vi "ServerTake2.vi"() -> ()   [LabVIEW 2021]
uses:
  86556008-d19e-4632-a649-a7f0de4e085f.vi
  5d9f77ae-4eb7-4624-8507-499cb33e88e0.vi
  9a779ec1-8874-4ed7-8bc4-c0cd389ef899.vi
  3957625e-ef2c-40df-94d6-cc40180103aa.vi
  b28d0b89-d437-4566-8e34-c46da29a0ee1.vi
  6f342689-c146-4fba-b3a6-fb699f7c09ee.vi
  <vilib>/Utility/file.llb/Write Delimited Spreadsheet (string).vi
panel:
  in  "file path (dialog if empty)":path=path "D:/APU Stuff/Bachelor of Computer Science (Intelligent Systems) [APD2F2202CS(IS)]/Semester 1/System Programming and Computer Control [CT047-3-2-SPCC]/Assignment/SystemRedo/Zone Status Changes.csv"
  in  "stop":bool
  in  "Tamper":cluster{u32, u32}[](array[cluster])
  in  "Alarm":cluster{u32, u32}[](array[cluster])
  in  "Bypass":cluster{u32, u32}[](array[cluster])
  in  "Normal":cluster{u32, u32}[](array[cluster])
  out "Zone 6":bool
  out "Zone 5":bool
  out "Zone 4":bool
  out "Zone 3":bool
  out "Zone 2":bool
  out "Zone 1":bool
  # "Green = Normal\nRed = Alarm\nOrange = Tamper\nBlue = Bypass"
  # "Zone Status Indicators"
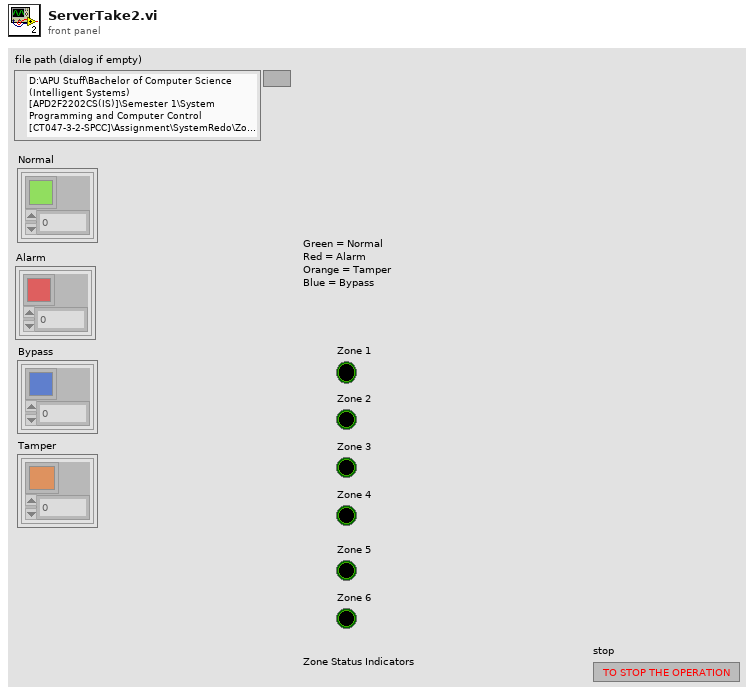
[diagram p1: front panel]
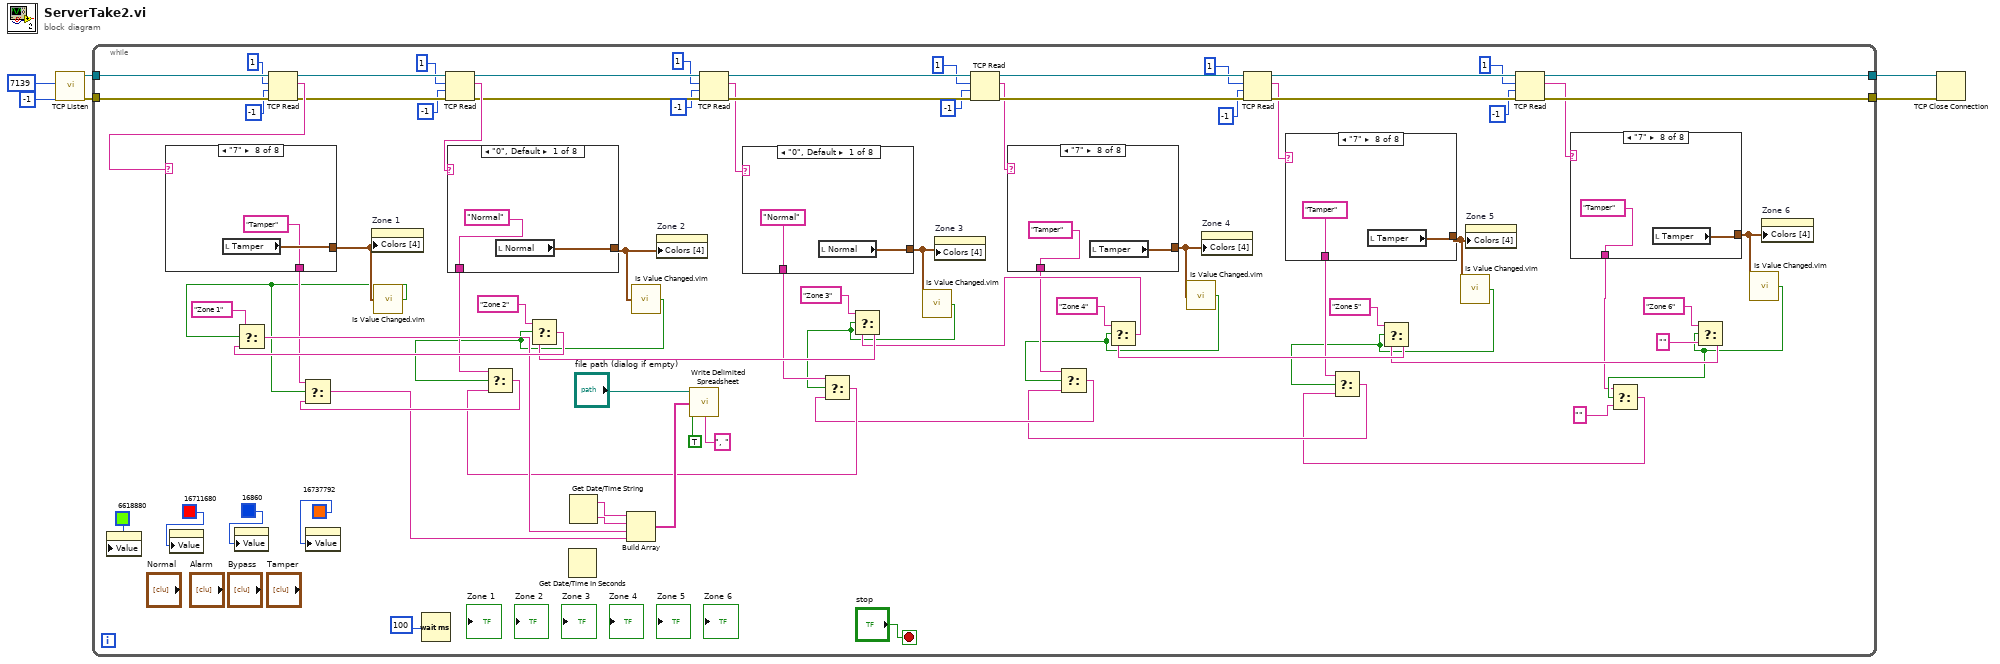
[diagram p0: block diagram]
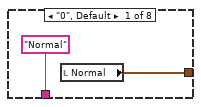
[diagram p2: hidden frame]
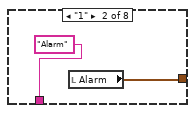
[diagram p3: hidden frame]
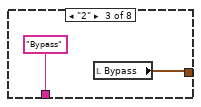
[diagram p4: hidden frame]
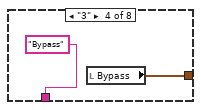
[diagram p5: hidden frame]
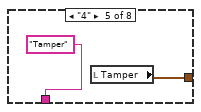
[diagram p6: hidden frame]
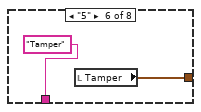
[diagram p7: hidden frame]
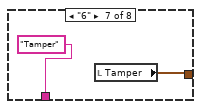
[diagram p8: hidden frame]
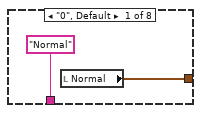
[diagram p9: hidden frame]
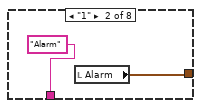
[diagram p10: hidden frame]
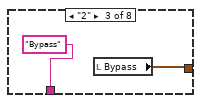
[diagram p11: hidden frame]
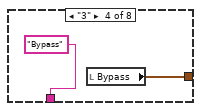
[diagram p12: hidden frame]
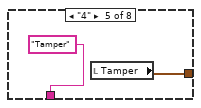
[diagram p13: hidden frame]
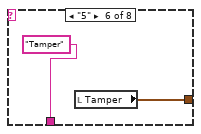
[diagram p14: hidden frame]
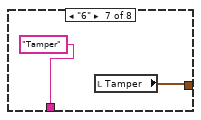
[diagram p15: hidden frame]
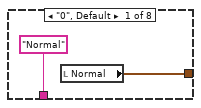
[diagram p16: hidden frame]
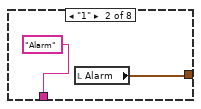
[diagram p17: hidden frame]
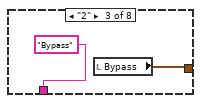
[diagram p18: hidden frame]
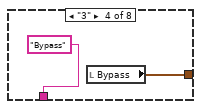
[diagram p19: hidden frame]
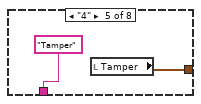
[diagram p20: hidden frame]
diagram:
  n1 = call <vilib>:"TCP Listen.vi"("timeout ms (wait forever: -1)"=-1, "port"=u16 7139) -> ("error out"=w2:errorcluster, "connection ID"=w4:refnum<k5>)  [unwired: 5 in, 3 out]
  n2 = while {
    tunnel: w4 -> [w88]
    tunnel: [w67] -> w3
    tunnel: w2 -> [w87]
    tunnel: [w63] -> w1
    stop <- "stop" stop-if-true
    n3 = property class="ColBox"("Value"=u32 6618880) -> ()  [unwired: 2 in, 2 out]
    n4 = property class="ColBox"("Value"=u32 16711680) -> ()  [unwired: 2 in, 2 out]
    n5 = property class="ColBox"("Value"=u32 16860) -> ()  [unwired: 2 in, 2 out]
    n6 = TCP Read(connection ID=w88, bytes to read=1, error in (no error)=w87, 9:-1 ("timeout ms (25000)")) -> (connection ID out=w77:refnum<k5>, data out=w84:string, error out=w76:errorcluster)  [unwired: 1 in]
    n7 = case shown="\"7\"" w84 {
      tunnel: [w170 w172 w174 w176 w178 w180 w182 w184] -> w41
      tunnel: ["Normal" "Alarm" "Bypass" "Bypass" "Tamper" "Tamper" "Tamper" "Tamper"] -> w25
      frame "0", Default {
        n8 = local read "Normal"() -> (w170:cluster{u32, u32}[])
      }
      frame "1" {
        n9 = local read "Alarm"() -> (w172:cluster{u32, u32}[])
      }
      frame "2" {
        n10 = local read "Bypass"() -> (w174:cluster{u32, u32}[])
      }
      frame "3" {
        n11 = local read "Bypass"() -> (w176:cluster{u32, u32}[])
      }
      frame "4" {
        n12 = local read "Tamper"() -> (w178:cluster{u32, u32}[])
      }
      frame "5" {
        n13 = local read "Tamper"() -> (w180:cluster{u32, u32}[])
      }
      frame "6" {
        n14 = local read "Tamper"() -> (w182:cluster{u32, u32}[])
      }
      frame "7" {
        n15 = local read "Tamper"() -> (w184:cluster{u32, u32}[])
      }
    }
    n16 = property class="ColBox"("Value"=u32 16737792) -> ()  [unwired: 2 in, 2 out]
    n17 = property on="Zone 1" class="Bool (strict)"("Colors [4]"=w41) -> ()  [unwired: 2 in, 2 out]
    n18 = call "Is Value Changed.vim"("value"=w41) -> ("changed or first call?"=w24:bool)
    n19 = Wait (ms)(milliseconds to wait=100) -> ()  [unwired: 1 out]
    n20 = TCP Read(connection ID=w77, bytes to read=1, error in (no error)=w76, 9:-1 ("timeout ms (25000)")) -> (connection ID out=w72:refnum<k5>, data out=w75:string, error out=w68:errorcluster)  [unwired: 1 in]
    n21 = case shown="\"0\", Default" w75 {
      tunnel: [w154 w156 w158 w160 w162 w164 w166 w168] -> w39
      tunnel: ["Normal" "Alarm" "Bypass" "Bypass" "Tamper" "Tamper" "Tamper" "Tamper"] -> w23
      frame "0", Default {
        n22 = local read "Normal"() -> (w154:cluster{u32, u32}[])
      }
      frame "1" {
        n23 = local read "Alarm"() -> (w156:cluster{u32, u32}[])
      }
      frame "2" {
        n24 = local read "Bypass"() -> (w158:cluster{u32, u32}[])
      }
      frame "3" {
        n25 = local read "Bypass"() -> (w160:cluster{u32, u32}[])
      }
      frame "4" {
        n26 = local read "Tamper"() -> (w162:cluster{u32, u32}[])
      }
      frame "5" {
        n27 = local read "Tamper"() -> (w164:cluster{u32, u32}[])
      }
      frame "6" {
        n28 = local read "Tamper"() -> (w166:cluster{u32, u32}[])
      }
      frame "7" {
        n29 = local read "Tamper"() -> (w168:cluster{u32, u32}[])
      }
    }
    n30 = Get Date/Time In Seconds() -> ()  [unwired: 1 out]
    n31 = Get Date/Time String() -> (date string=w49:string, time string=w48:string)  [unwired: 3 in]
    n32 = call "Is Value Changed.vim"("value"=w39) -> ("changed or first call?"=w22:bool)
    n33 = property on="Zone 2" class="Bool (strict)"("Colors [4]"=w39) -> ()  [unwired: 2 in, 2 out]
    n34 = TCP Read(connection ID=w72, bytes to read=1, error in (no error)=w68, 9:-1 ("timeout ms (25000)")) -> (connection ID out=w71:refnum<k5>, data out=w54:string, error out=w66:errorcluster)  [unwired: 1 in]
    n35 = case shown="\"0\", Default" w54 {
      tunnel: [w138 w140 w142 w144 w146 w148 w150 w152] -> w38
      tunnel: ["Normal" "Alarm" "Bypass" "Bypass" "Tamper" "Tamper" "Tamper" "Tamper"] -> w19
      frame "0", Default {
        n36 = local read "Normal"() -> (w138:cluster{u32, u32}[])
      }
      frame "1" {
        n37 = local read "Alarm"() -> (w140:cluster{u32, u32}[])
      }
      frame "2" {
        n38 = local read "Bypass"() -> (w142:cluster{u32, u32}[])
      }
      frame "3" {
        n39 = local read "Bypass"() -> (w144:cluster{u32, u32}[])
      }
      frame "4" {
        n40 = local read "Tamper"() -> (w146:cluster{u32, u32}[])
      }
      frame "5" {
        n41 = local read "Tamper"() -> (w148:cluster{u32, u32}[])
      }
      frame "6" {
        n42 = local read "Tamper"() -> (w150:cluster{u32, u32}[])
      }
      frame "7" {
        n43 = local read "Tamper"() -> (w152:cluster{u32, u32}[])
      }
    }
    n44 = call "Is Value Changed.vim"("value"=w38) -> ("changed or first call?"=w17:bool)
    n45 = property on="Zone 3" class="Bool (strict)"("Colors [4]"=w38) -> ()  [unwired: 2 in, 2 out]
    n46 = TCP Read(connection ID=w71, bytes to read=1, error in (no error)=w66, 9:-1 ("timeout ms (25000)")) -> (connection ID out=w70:refnum<k5>, data out=w51:string, error out=w65:errorcluster)  [unwired: 1 in]
    n47 = case shown="\"7\"" w51 {
      tunnel: [w122 w124 w126 w128 w130 w132 w134 w136] -> w35
      tunnel: ["Normal" "Alarm" "Bypass" "Bypass" "Tamper" "Tamper" "Tamper" "Tamper"] -> w16
      frame "0", Default {
        n48 = local read "Normal"() -> (w122:cluster{u32, u32}[])
      }
      frame "1" {
        n49 = local read "Alarm"() -> (w124:cluster{u32, u32}[])
      }
      frame "2" {
        n50 = local read "Bypass"() -> (w126:cluster{u32, u32}[])
      }
      frame "3" {
        n51 = local read "Bypass"() -> (w128:cluster{u32, u32}[])
      }
      frame "4" {
        n52 = local read "Tamper"() -> (w130:cluster{u32, u32}[])
      }
      frame "5" {
        n53 = local read "Tamper"() -> (w132:cluster{u32, u32}[])
      }
      frame "6" {
        n54 = local read "Tamper"() -> (w134:cluster{u32, u32}[])
      }
      frame "7" {
        n55 = local read "Tamper"() -> (w136:cluster{u32, u32}[])
      }
    }
    n56 = call "Is Value Changed.vim"("value"=w35) -> ("changed or first call?"=w15:bool)
    n57 = property on="Zone 4" class="Bool (strict)"("Colors [4]"=w35) -> ()  [unwired: 2 in, 2 out]
    n58 = TCP Read(connection ID=w70, bytes to read=1, error in (no error)=w65, 9:-1 ("timeout ms (25000)")) -> (connection ID out=w69:refnum<k5>, data out=w52:string, error out=w64:errorcluster)  [unwired: 1 in]
    n59 = case shown="\"7\"" w52 {
      tunnel: [w106 w108 w110 w112 w114 w116 w118 w120] -> w36
      tunnel: ["Normal" "Alarm" "Bypass" "Bypass" "Tamper" "Tamper" "Tamper" "Tamper"] -> w13
      frame "0", Default {
        n60 = local read "Normal"() -> (w106:cluster{u32, u32}[])
      }
      frame "1" {
        n61 = local read "Alarm"() -> (w108:cluster{u32, u32}[])
      }
      frame "2" {
        n62 = local read "Bypass"() -> (w110:cluster{u32, u32}[])
      }
      frame "3" {
        n63 = local read "Bypass"() -> (w112:cluster{u32, u32}[])
      }
      frame "4" {
        n64 = local read "Tamper"() -> (w114:cluster{u32, u32}[])
      }
      frame "5" {
        n65 = local read "Tamper"() -> (w116:cluster{u32, u32}[])
      }
      frame "6" {
        n66 = local read "Tamper"() -> (w118:cluster{u32, u32}[])
      }
      frame "7" {
        n67 = local read "Tamper"() -> (w120:cluster{u32, u32}[])
      }
    }
    n68 = call "Is Value Changed.vim"("value"=w36) -> ("changed or first call?"=w11:bool)
    n69 = property on="Zone 5" class="Bool (strict)"("Colors [4]"=w36) -> ()  [unwired: 2 in, 2 out]
    n70 = TCP Read(connection ID=w69, bytes to read=1, error in (no error)=w64, 9:-1 ("timeout ms (25000)")) -> (connection ID out=w67:refnum<k5>, data out=w53:string, error out=w63:errorcluster)  [unwired: 1 in]
    n71 = case shown="\"7\"" w53 {
      tunnel: [w90 w92 w94 w96 w98 w100 w102 w104] -> w37
      tunnel: ["Normal" "Alarm" "Bypass" "Bypass" "Tamper" "Tamper" "Tamper" "Tamper"] -> w7
      frame "0", Default {
        n72 = local read "Normal"() -> (w90:cluster{u32, u32}[])
      }
      frame "1" {
        n73 = local read "Alarm"() -> (w92:cluster{u32, u32}[])
      }
      frame "2" {
        n74 = local read "Bypass"() -> (w94:cluster{u32, u32}[])
      }
      frame "3" {
        n75 = local read "Bypass"() -> (w96:cluster{u32, u32}[])
      }
      frame "4" {
        n76 = local read "Tamper"() -> (w98:cluster{u32, u32}[])
      }
      frame "5" {
        n77 = local read "Tamper"() -> (w100:cluster{u32, u32}[])
      }
      frame "6" {
        n78 = local read "Tamper"() -> (w102:cluster{u32, u32}[])
      }
      frame "7" {
        n79 = local read "Tamper"() -> (w104:cluster{u32, u32}[])
      }
    }
    n80 = call "Is Value Changed.vim"("value"=w37) -> ("changed or first call?"=w8:bool)
    n81 = Select(t=w7, s=w8, f="") -> (s? t:f=w10:string)
    n82 = Select(t=w13, s=w11, f=w10) -> (s? t:f=w12:string)
    n83 = Select(t=w16, s=w15, f=w12) -> (s? t:f=w14:string)
    n84 = Select(t=w19, s=w17, f=w14) -> (s? t:f=w18:string)
    n85 = Select(t=w23, s=w22, f=w18) -> (s? t:f=w21:string)
    n86 = Select(t=w25, s=w24, f=w21) -> (s? t:f=w20:string)
    n87 = Select(t="Zone 6", s=w8, f="") -> (s? t:f=w27:string)
    n88 = Select(t="Zone 5", s=w11, f=w27) -> (s? t:f=w28:string)
    n89 = Select(t="Zone 4", s=w15, f=w28) -> (s? t:f=w29:string)
    n90 = Select(t="Zone 3", s=w17, f=w29) -> (s? t:f=w30:string)
    n91 = Select(t="Zone 2", s=w22, f=w30) -> (s? t:f=w42:string)
    n92 = Select(t="Zone 1", s=w24, f=w42) -> (s? t:f=w40:string)
    n93 = Build Array(w49, w48, w40, w20) -> (w47:string[])
    n94 = call-poly <vilib>:"Write Delimited Spreadsheet.vi"("file path (dialog if empty)"="file path (dialog if empty)", "1D data"=w47, "append to file? (new file:F)"=TRUE, "delimiter (\\t)"=", " ("delimiter (\\t)")) -> ()  [unwired: 10 in, 2 out]
    n95 = property on="Zone 6" class="Bool (strict)"("Colors [4]"=w37) -> ()  [unwired: 2 in, 2 out]
  }
  n96 = TCP Close Connection(connection ID=w3, error in (no error)=w1) -> ()  [unwired: 1 in, 2 out]
